vi "Set Header Object Positions.vi"(4 "FP.width":i16, 8 "error in":errorcluster, 10 "label array in":string[](array[string]), 11 "controls[] in":refnum<vi>[](array[refnum])) -> (0 "error out":errorcluster, 2 "label array out":string[](array[string]), 3 "controls[] out":refnum<vi>[](array[refnum]))   [LabVIEW 2018]
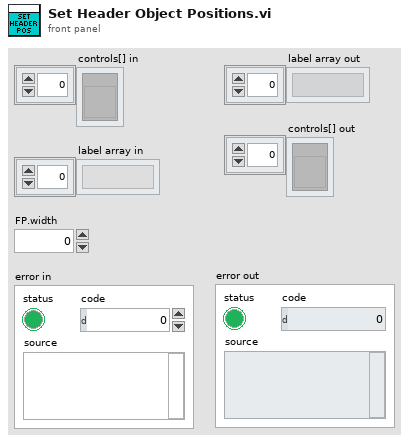
[diagram p1: front panel]
types:
  T1 = typedef "LVRectTypeDef.ctl" = cluster{"Left":i16, "Top":i16, "Right":i16, "Bottom":i16}
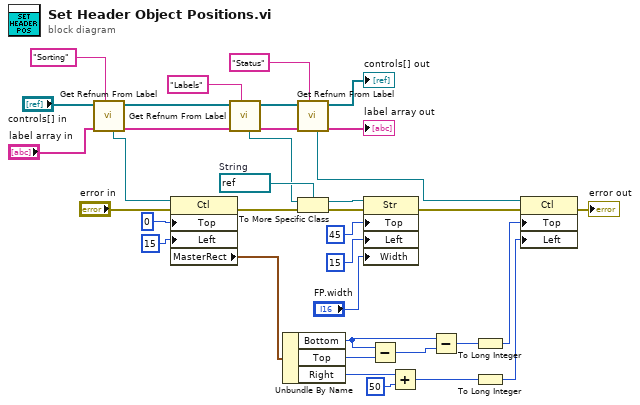
[diagram p0: block diagram]
diagram:
  w28 = refnum<vi> refnum  # String
  n1 = call "Get Refnum From Label.vi"("label"="Sorting" ("element"), "label array in"="label array in", "controls[] in"="controls[] in") -> ("label array out"=w9:string[], "controls[] out"=w8:refnum<vi>[], "refnum out"=w10:refnum<vi>)  [unwired: 6 in]
  n2 = property class="Ctl"(reference=w10, error in="error in", "Top"=0 ("Position:Left"), "Left"=15 ("Position:Top")) -> (error out=w31:errorcluster, "MasterRect"=w23:T1)  [unwired: 1 out]
  n3 = call "Get Refnum From Label.vi"("label"="Labels" ("element"), "label array in"=w9, "controls[] in"=w8) -> ("label array out"=w33:string[], "controls[] out"=w34:refnum<vi>[], "refnum out"=w27:refnum<vi>)  [unwired: 6 in]
  n4 = Unbundle By Name(w23) -> ("Bottom"=w24:i16, "Top"=w16:i16, "Right"=w18:i16)
  n5 = call "Get Refnum From Label.vi"("label"="Status", "label array in"=w33, "controls[] in"=w34) -> ("label array out"=→"label array out":string[], "controls[] out"=→"controls[] out":refnum<vi>[], "refnum out"=w17:refnum<vi>)  [unwired: 6 in]
  n6 = To More Specific Class(target class=w28, reference=w27, error in=w31) -> (specific class reference=w29:refnum<vi>, error out=w32:errorcluster)
  n7 = property class="Str"(reference=w29, error in=w32, "Top"=45 ("Position:Top"), "Left"=15 ("Position:Left"), "Width"="FP.width") -> (error out=w2:errorcluster)  [unwired: 1 out]
  n8 = Subtract(x=w24, y=w16) -> (x-y=w25:i16)
  n9 = Add(x=w18, y=i16 50) -> (x+y=w21:i16)
  n10 = Subtract(x=w24, y=w25) -> (x-y=w26:i16)
  n11 = To Long Integer(number=w26) -> (32bit integer=w19:i32)
  n12 = To Long Integer(number=w21) -> (32bit integer=w20:i32)
  n13 = property class="Ctl"(reference=w17, error in=w2, "Top"=w19, "Left"=w20) -> (error out=→"error out":errorcluster)  [unwired: 1 out]
